vi "PicoScope6000AdvancedTriggerSettings.vi"(0 "handle in":i16, 1 "Channel A Trigger Properties":T1={"thresholdUpper"=0, "thresholdUpperHysteresis"=0, "thresholdLower"=0, "thresholdLowerHysteresis"=0, "Threshold Mode"=0, "Direction"=0, "Available"=TRUE} {"Direction" items=["Above / Inside", "Below / Outside", "Rising / Enter", "Falling / Exit", "Rising or Falling / Enter or Exit", "Above Lower", "Below Lower", "Rising Lower", "Falling Lower", "Positive Runt", "Negative Runt"]; "Threshold Mode" items=["Level", "Window"]}, 2 "Channel B Trigger Properties":T1={"thresholdUpper"=0, "thresholdUpperHysteresis"=0, "thresholdLower"=0, "thresholdLowerHysteresis"=0, "Threshold Mode"=0, "Direction"=0, "Available"=TRUE} {"Direction" items=["Above / Inside", "Below / Outside", "Rising / Enter", "Falling / Exit", "Rising or Falling / Enter or Exit", "Above Lower", "Below Lower", "Rising Lower", "Falling Lower", "Positive Runt", "Negative Runt"]; "Threshold Mode" items=["Level", "Window"]}, 3 "Channel C Trigger Properties":T1 {"Direction" items=["Above / Inside", "Below / Outside", "Rising / Enter", "Falling / Exit", "Rising or Falling / Enter or Exit", "Above Lower", "Below Lower", "Rising Lower", "Falling Lower", "Positive Runt", "Negative Runt"]; "Threshold Mode" items=["Level", "Window"]}, 5 "Auto Trigger (ms)":i32, 7 "Trigger Conditions":T4 {"Condition Logic" items=["AND", "OR", "XOR"]}, 8 "Pulse Width Qualifier Settings":T2={"Direction"=2, "Lower Limit"=0, "Upper Limit"=0, "Pulse Width Type"=4} {"Pulse Width Type" items=["None", "Less Than", "Greater Than", "In Range", "Out of Range"]; "Direction" items=["Rising"=2, "Falling"=3, "Rising Lower"=7, "Falling Lower"=8]}, 9 "Trigger Delay":u32, 10 "Pulse Width Qualifier Conditions":T3 {"Condition Logic" items=["AND", "OR", "XOR"]}, 11 "error in":errorcluster, 12 "Channel D Trigger Properties":T1 {"Direction" items=["Above / Inside", "Below / Outside", "Rising / Enter", "Falling / Exit", "Rising or Falling / Enter or Exit", "Above Lower", "Below Lower", "Rising Lower", "Falling Lower", "Positive Runt", "Negative Runt"]; "Threshold Mode" items=["Level", "Window"]}, 13 "Ext. Trigger Properties":T1 {"Direction" items=["Above / Inside", "Below / Outside", "Rising / Enter", "Falling / Exit", "Rising or Falling / Enter or Exit", "Above Lower", "Below Lower", "Rising Lower", "Falling Lower", "Positive Runt", "Negative Runt"]; "Threshold Mode" items=["Level", "Window"]}, 14 "Aux. Trigger Properties":T1 {"Direction" items=["Above / Inside", "Below / Outside", "Rising / Enter", "Falling / Exit", "Rising or Falling / Enter or Exit", "Above Lower", "Below Lower", "Rising Lower", "Falling Lower", "Positive Runt", "Negative Runt"]; "Threshold Mode" items=["Level", "Window"]}) -> (4 "handle out":i16, 15 "error out":errorcluster)   [LabVIEW 2010]
doc: "This VI is an interface for the advanced trigger features of the oscilloscope (a simple trigger can be set using PicoScope4000Settings.vi, in which case it is not necessary to use this VI)."
uses:
  ps6000.dll
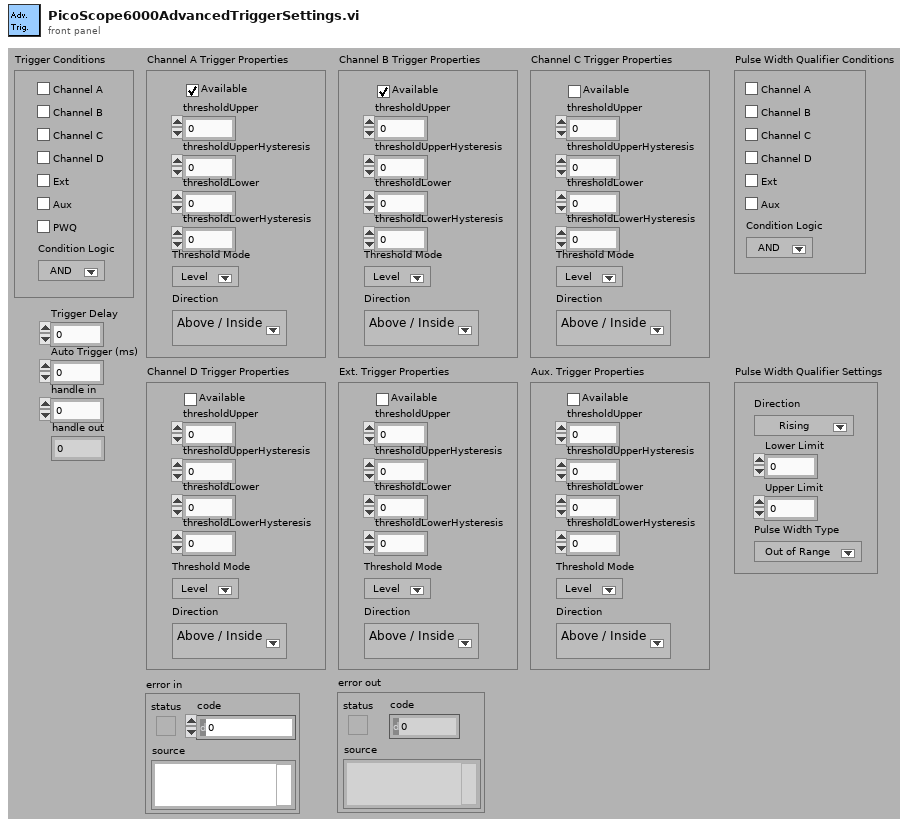
[diagram p1: front panel]
types:
  T1 = cluster{"thresholdUpper":i16, "thresholdUpperHysteresis":u16, "thresholdLower":i16, "thresholdLowerHysteresis":u16, "Threshold Mode":i32, "Direction":i32, "Available":bool}
  T2 = cluster{"Direction":i32, "Lower Limit":u32, "Upper Limit":u32, "Pulse Width Type":i32}
  T3 = cluster{"Channel A":bool, "Channel B":bool, "Channel C":bool, "Channel D":bool, "Aux":bool, "Condition Logic":u16, "Ext":bool}
  T4 = cluster{"Channel A":bool, "Channel B":bool, "Channel C":bool, "Channel D":bool, "Aux":bool, "PWQ":bool, "Condition Logic":u16, "Ext":bool}
  T5 = cluster{"thresholdUpper":i16, "thresholdUpperHysteresis":u16, "thresholdLower":i16, "thresholdLowerHysteresis":u16, "Threshold Mode":i32, "Direction":i32, "Available":bool}[]
  T6 = cluster{"[0]":i32, "[1]":i32, "[2]":i32, "[3]":i32, "[4]":i32, "[5]":i32, "[6]":i32, "[7]":i32, "[8]":i32}
  T7 = cluster{"status":bool, "code":u32, "source":string}
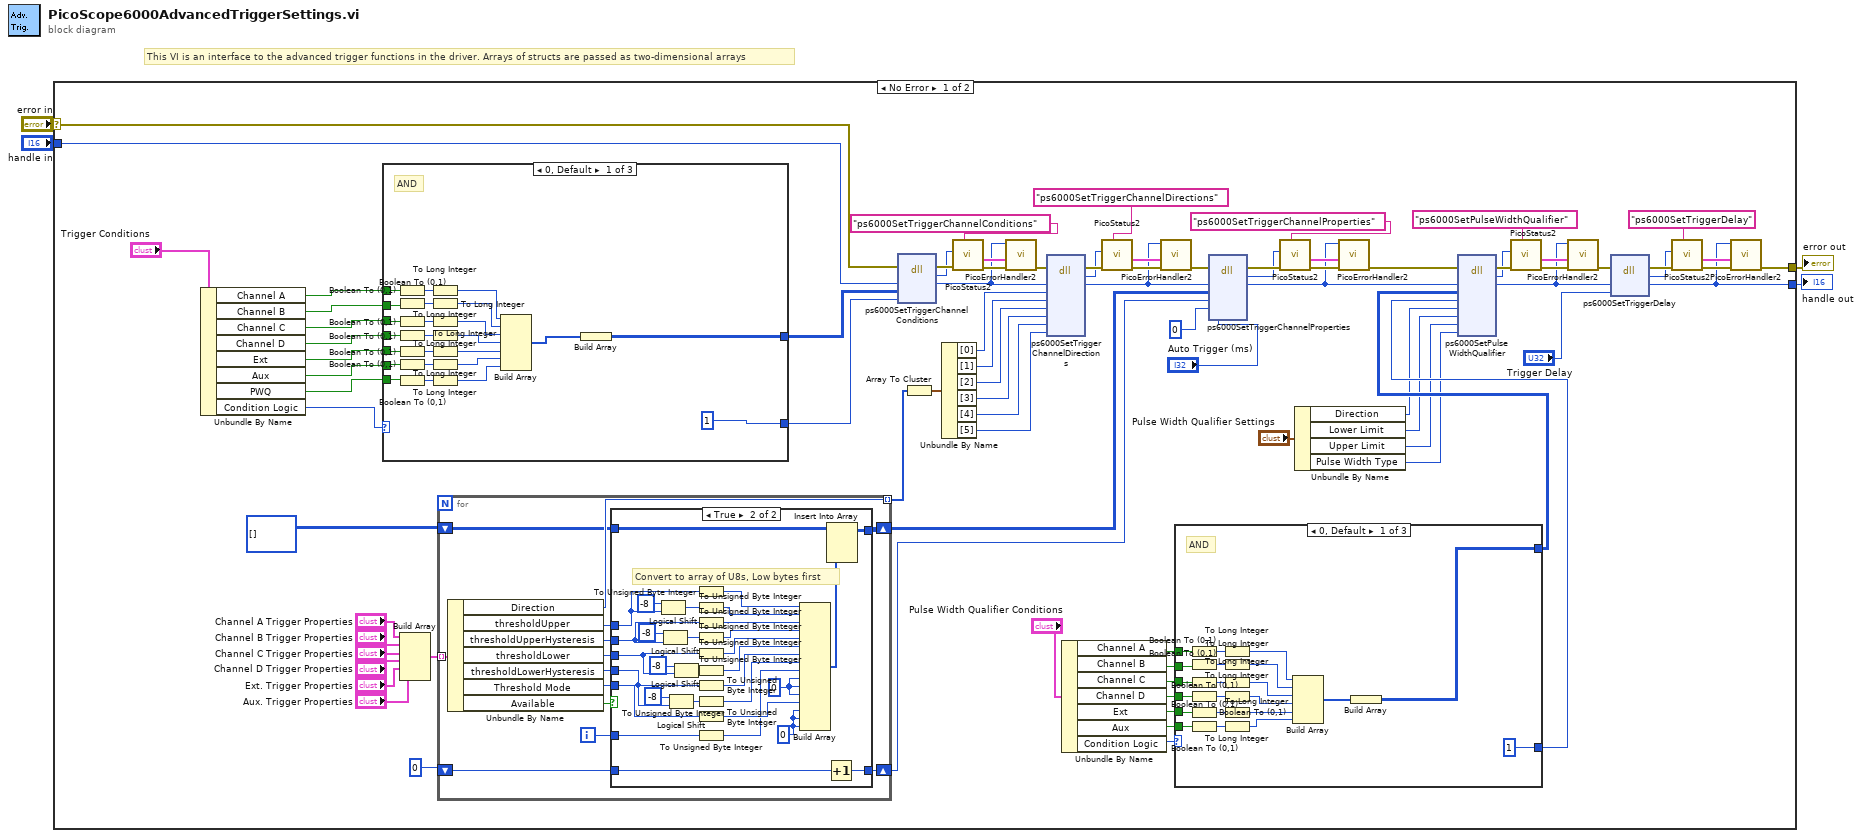
[diagram p0: block diagram]
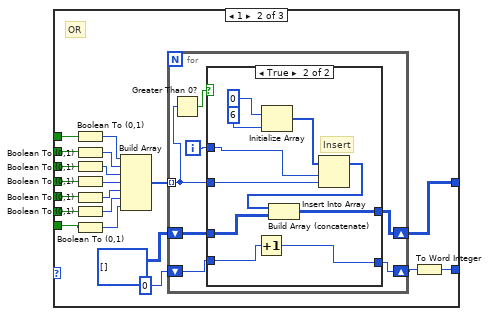
[diagram p2: hidden frame]
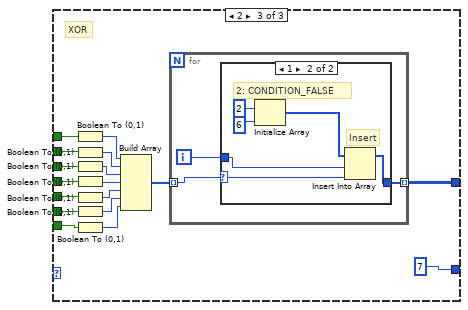
[diagram p4: hidden frame]
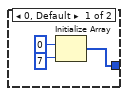
[diagram p5: hidden frame]
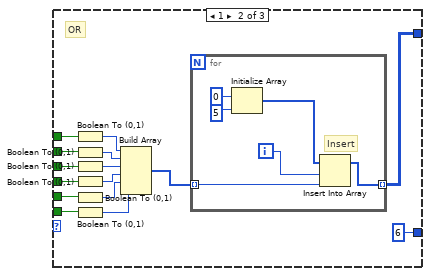
[diagram p6: hidden frame]
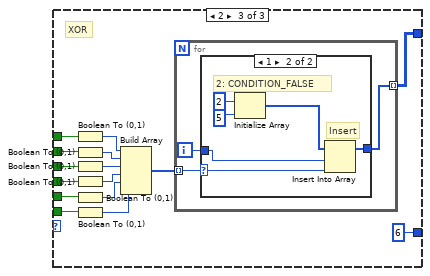
[diagram p7: hidden frame]
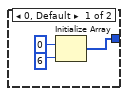
[diagram p8: hidden frame]
diagram:
  # "This VI is an interface to the advanced trigger functions in the driver. Arrays of structs are passed as two-dimensional arrays"
  n1 = case shown="No Error" "error in" {
    selector: "error in" -> [w54 w297]
    tunnel: "handle in" -> [w55 w298]
    tunnel: [w35 w298] -> w2
    tunnel: [w36 w297] -> w1
    frame No Error {
      n2 = Unbundle By Name("Trigger Conditions") -> ("Channel A"=w49:bool, "Channel B"=w48:bool, "Channel C"=w47:bool, "Channel D"=w46:bool, "Ext"=w45:bool, "Aux"=w44:bool, "PWQ"=w43:bool, "Condition Logic"=w40:u16)
      n3 = case shown="0, Default" w40 {
        tunnel: w49 -> [w113 w133 w169]
        tunnel: w48 -> [w105 w132 w168]
        tunnel: w47 -> [w104 w131 w167]
        tunnel: w46 -> [w103 w130 w166]
        tunnel: w45 -> [w102 w129 w165]
        tunnel: w44 -> [w101 w128 w164]
        tunnel: [w92 w119 w155] -> w41
        tunnel: [i16 1 w115 i16 7] -> w42
        tunnel: w43 -> [w90 w116 w153]
        frame 0, Default {
          # "AND"
          n4 = Boolean To (0,1)(Boolean=w113) -> (0, 1=w112:i16)
          n5 = Boolean To (0,1)(Boolean=w105) -> (0, 1=w111:i16)
          n6 = Boolean To (0,1)(Boolean=w104) -> (0, 1=w110:i16)
          n7 = Boolean To (0,1)(Boolean=w103) -> (0, 1=w109:i16)
          n8 = Boolean To (0,1)(Boolean=w102) -> (0, 1=w108:i16)
          n9 = Boolean To (0,1)(Boolean=w101) -> (0, 1=w107:i16)
          n10 = Boolean To (0,1)(Boolean=w90) -> (0, 1=w106:i16)
          n11 = To Long Integer(number=w112) -> (32bit integer=w100:i32)
          n12 = To Long Integer(number=w111) -> (32bit integer=w99:i32)
          n13 = To Long Integer(number=w110) -> (32bit integer=w98:i32)
          n14 = To Long Integer(number=w109) -> (32bit integer=w97:i32)
          n15 = To Long Integer(number=w108) -> (32bit integer=w96:i32)
          n16 = To Long Integer(number=w107) -> (32bit integer=w95:i32)
          n17 = To Long Integer(number=w106) -> (32bit integer=w94:i32)
          n18 = Build Array(w100, w99, w98, w97, w96, w95, w94) -> (w93:i32[])
          n19 = Build Array(w93) -> (w92:i32[][])
        }
        frame 1 {
          # "OR"
          n20 = Boolean To (0,1)(Boolean=w133) -> (0, 1=w121:i16)
          n21 = Boolean To (0,1)(Boolean=w132) -> (0, 1=w122:i16)
          n22 = Boolean To (0,1)(Boolean=w131) -> (0, 1=w123:i16)
          n23 = Boolean To (0,1)(Boolean=w130) -> (0, 1=w124:i16)
          n24 = Boolean To (0,1)(Boolean=w129) -> (0, 1=w125:i16)
          n25 = Boolean To (0,1)(Boolean=w128) -> (0, 1=w126:i16)
          n26 = Boolean To (0,1)(Boolean=w116) -> (0, 1=w127:i16)
          n27 = Build Array(w121, w122, w123, w124, w125, w126, w127) -> (w120:i16[])
          n28 = for {
            tunnel: w120 -> [w137] mode=indexing
            shift-right: [w136] -> w119
            shift-left: i32[][] [] -> [w140]
            shift-right: [w134] -> w114
            shift-left: 0 -> [w135]
            i -> [w139]
            n29 = Greater Than 0?(x=w137) -> (x > 0?=w138:bool)
            n30 = case shown="True" w138 {
              tunnel: w140 -> [w142 w145]
              tunnel: w139 -> [_ w149]
              tunnel: w137 -> [_ w148]
              tunnel: [w142 w147] -> w136
              tunnel: w135 -> [w141 w144]
              tunnel: [w141 w143] -> w134
              frame False {
              }
              frame True {
                # "Insert"
                n31 = Increment(x=w144) -> (x+1=w143:i32)
                n32 = Initialize Array(0 ("element"), 6 ("dimension size")) -> (w150:i32[])
                n33 = Insert Into Array(array=w150, index=w149, new element=w148) -> (w146:i32[])
                n34 = Build Array (concatenate)(w146, w145) -> (w147:i32[][])
              }
            }
          }
          n35 = To Word Integer(number=w114) -> (16bit integer=w115:i16)
        }
        frame 2 {
          # "XOR"
          n36 = Boolean To (0,1)(Boolean=w169) -> (0, 1=w157:i16)
          n37 = Boolean To (0,1)(Boolean=w168) -> (0, 1=w158:i16)
          n38 = Boolean To (0,1)(Boolean=w167) -> (0, 1=w159:i16)
          n39 = Boolean To (0,1)(Boolean=w166) -> (0, 1=w160:i16)
          n40 = Boolean To (0,1)(Boolean=w165) -> (0, 1=w161:i16)
          n41 = Boolean To (0,1)(Boolean=w164) -> (0, 1=w162:i16)
          n42 = Boolean To (0,1)(Boolean=w153) -> (0, 1=w163:i16)
          n43 = Build Array(w157, w158, w159, w160, w161, w162, w163) -> (w156:i16[])
          n44 = for {
            tunnel: w156 -> [w170] mode=indexing
            tunnel: [w172] -> w155 mode=indexing
            i -> [w171]
            n45 = case shown="1" w170 {
              selector: w170 -> [_ w177]
              tunnel: [w173 w178] -> w172
              tunnel: w171 -> [_ w176]
              frame 0, Default {
                n46 = Initialize Array(0 ("element"), 7 ("dimension size")) -> (w173:i32[])
              }
              frame 1 {
                # "2: CONDITION_FALSE"
                # "Insert"
                n47 = Initialize Array(2 ("element"), 6 ("dimension size")) -> (w179:i32[])
                n48 = Insert Into Array(array=w179, index=w176, new element=w177) -> (w178:i32[])
              }
            }
          }
        }
      }
      n49 = Build Array("Channel A Trigger Properties", "Channel B Trigger Properties", "Channel C Trigger Properties", "Channel D Trigger Properties", "Ext. Trigger Properties", "Aux. Trigger Properties") -> (w85:T5)
      n50 = for {
        tunnel: w85 -> [w258] mode=indexing
        tunnel: [w257] -> w84 mode=indexing
        shift-right: [w254] -> w52
        shift-left: i16 0 -> [w253]
        shift-right: [w251] -> w50
        shift-left: u8[][] [] -> [w252]
        i -> [w255]
        n51 = Unbundle By Name(w258) -> ("Direction"=w257:i32, "thresholdUpper"=w263:i16, "thresholdUpperHysteresis"=w262:u16, "thresholdLower"=w261:i16, "thresholdLowerHysteresis"=w260:u16, "Threshold Mode"=w259:i32, "Available"=w256:bool)
        n52 = case shown="True" w256 {
          tunnel: w263 -> [_ w295]
          tunnel: w262 -> [_ w287]
          tunnel: w261 -> [_ w286]
          tunnel: w260 -> [_ w285]
          tunnel: w259 -> [_ w276]
          tunnel: w255 -> [_ w271]
          tunnel: [w265 w270] -> w254
          tunnel: w253 -> [w265 w269]
          tunnel: [w264 w267] -> w251
          tunnel: w252 -> [w264 w266]
          frame False {
          }
          frame True {
            w274 = u8 0 ("element")
            w275 = u8 0 ("element")
            # "Convert to array of U8s, Low bytes first"
            n53 = Logical Shift(y=i16 -8, x=w295) -> (x << y=w294:i16)
            n54 = Logical Shift(y=i16 -8, x=w287) -> (x << y=w293:u16)
            n55 = Logical Shift(y=i16 -8, x=w285) -> (x << y=w289:u16)
            n56 = Logical Shift(y=i16 -8, x=w286) -> (x << y=w290:i16)
            n57 = To Unsigned Byte Integer(number=w295) -> (unsigned 8bit integer=w284:u8)
            n58 = To Unsigned Byte Integer(number=w294) -> (unsigned 8bit integer=w283:u8)
            n59 = To Unsigned Byte Integer(number=w287) -> (unsigned 8bit integer=w282:u8)
            n60 = To Unsigned Byte Integer(number=w293) -> (unsigned 8bit integer=w281:u8)
            n61 = To Unsigned Byte Integer(number=w286) -> (unsigned 8bit integer=w280:u8)
            n62 = To Unsigned Byte Integer(number=w290) -> (unsigned 8bit integer=w279:u8)
            n63 = To Unsigned Byte Integer(number=w285) -> (unsigned 8bit integer=w278:u8)
            n64 = To Unsigned Byte Integer(number=w289) -> (unsigned 8bit integer=w277:u8)
            n65 = To Unsigned Byte Integer(number=w276) -> (unsigned 8bit integer=w273:u8)
            n66 = To Unsigned Byte Integer(number=w271) -> (unsigned 8bit integer=w272:u8)
            n67 = Build Array(w284, w283, w282, w281, w280, w279, w278, w277, w272, w275, w275, w275, w273, w274, w274, w274) -> (w268:u8[])
            n68 = Increment(x=w269) -> (x+1=w270:i16)
            n69 = Insert Into Array(array=w266, new element=w268) -> (w267:u8[][])  [unwired: 2 in]
          }
        }
      }
      n70 = dll-call lib="PS6000.dll" fn="ps6000SetTriggerChannelConditions" ("ps3000.dll:_ps3000_open_unit@0")(error in=w54, "handle"=w55, "conditions"=w41, "nConditions"=w42) -> (error out=w20:errorcluster, "PICO_STATUS"=w9:u32, "handle"=w10:i16)  [unwired: 4 in, 1 out]
      n71 = Array To Cluster(array=w84) -> (cluster=w83:T6)
      n72 = Unbundle By Name(w83) -> ("[0]"=w82:i32, "[1]"=w81:i32, "[2]"=w80:i32, "[3]"=w79:i32, "[4]"=w78:i32, "[5]"=w77:i32)
      n73 = call "PicoStatus2.vi"("PICO source"="ps6000SetTriggerChannelConditions" ("source"), "Error in"=w20, "PICO STATUS"=w9) -> ("error out"=w22:errorcluster, "PICO_STATUS out"=w21:T7)  [unwired: 5 in]
      n74 = call "PicoErrorHandler2.vi"("error in (no error)"=w22, "PICO_STATUS in"=w21, "handle In"=w10) -> ("error out"=w19:errorcluster)  [unwired: 8 in]
      n75 = dll-call lib="PS6000.dll" fn="ps6000SetTriggerChannelDirections" ("ps3000.dll:_ps3000_open_unit@0")(error in=w19, "handle"=w10, "channelA"=w82, "channelB"=w81, "channelC"=w80, "channelD"=w79, "ext"=w78, "aux"=w77) -> (error out=w18:errorcluster, "PICO_STATUS"=w11:u32, "handle"=w12:i16)  [unwired: 8 in, 1 out]
      n76 = Unbundle By Name("Pulse Width Qualifier Conditions") -> ("Channel A"=w74:bool, "Channel B"=w73:bool, "Channel C"=w72:bool, "Channel D"=w71:bool, "Ext"=w70:bool, "Aux"=w61:bool, "Condition Logic"=w62:u16)
      n77 = call "PicoStatus2.vi"("PICO source"="ps6000SetTriggerChannelDirections" ("source"), "Error in"=w18, "PICO STATUS"=w11) -> ("error out"=w24:errorcluster, "PICO_STATUS out"=w23:T7)  [unwired: 5 in]
      n78 = call "PicoErrorHandler2.vi"("error in (no error)"=w24, "PICO_STATUS in"=w23, "handle In"=w12) -> ("error out"=w17:errorcluster)  [unwired: 8 in]
      n79 = case shown="0, Default" w62 {
        tunnel: w74 -> [w202 w217 w238]
        tunnel: w73 -> [w196 w216 w237]
        tunnel: w72 -> [w195 w215 w236]
        tunnel: w71 -> [w194 w214 w235]
        tunnel: w70 -> [w193 w205 w226]
        tunnel: [w186 w207 w228] -> w69
        tunnel: [i16 1 i16 6 i16 6] -> w68
        tunnel: w61 -> [w183 w204 w225]
        frame 0, Default {
          # "AND"
          n80 = Boolean To (0,1)(Boolean=w202) -> (0, 1=w201:i16)
          n81 = Boolean To (0,1)(Boolean=w196) -> (0, 1=w200:i16)
          n82 = Boolean To (0,1)(Boolean=w195) -> (0, 1=w199:i16)
          n83 = Boolean To (0,1)(Boolean=w194) -> (0, 1=w198:i16)
          n84 = Boolean To (0,1)(Boolean=w193) -> (0, 1=w197:i16)
          n85 = Boolean To (0,1)(Boolean=w183) -> (0, 1=w184:i16)
          n86 = To Long Integer(number=w201) -> (32bit integer=w192:i32)
          n87 = To Long Integer(number=w200) -> (32bit integer=w191:i32)
          n88 = To Long Integer(number=w199) -> (32bit integer=w190:i32)
          n89 = To Long Integer(number=w198) -> (32bit integer=w189:i32)
          n90 = To Long Integer(number=w197) -> (32bit integer=w188:i32)
          n91 = To Long Integer(number=w184) -> (32bit integer=w182:i32)
          n92 = Build Array(w192, w191, w190, w189, w188, w182) -> (w187:i32[])
          n93 = Build Array(w187) -> (w186:i32[][])
        }
        frame 1 {
          # "OR"
          n94 = Boolean To (0,1)(Boolean=w217) -> (0, 1=w209:i16)
          n95 = Boolean To (0,1)(Boolean=w216) -> (0, 1=w210:i16)
          n96 = Boolean To (0,1)(Boolean=w215) -> (0, 1=w211:i16)
          n97 = Boolean To (0,1)(Boolean=w214) -> (0, 1=w212:i16)
          n98 = Boolean To (0,1)(Boolean=w205) -> (0, 1=w213:i16)
          n99 = Boolean To (0,1)(Boolean=w204) -> (0, 1=w203:i16)
          n100 = Build Array(w209, w210, w211, w212, w213, w203) -> (w208:i16[])
          n101 = for {
            tunnel: w208 -> [w219] mode=indexing
            tunnel: [w218] -> w207 mode=indexing
            i -> [w220]
            # "Insert"
            n102 = Initialize Array(0 ("element"), 5 ("dimension size")) -> (w221:i32[])
            n103 = Insert Into Array(array=w221, index=w220, new element=w219) -> (w218:i32[])
          }
        }
        frame 2 {
          # "XOR"
          n104 = Boolean To (0,1)(Boolean=w238) -> (0, 1=w230:i16)
          n105 = Boolean To (0,1)(Boolean=w237) -> (0, 1=w231:i16)
          n106 = Boolean To (0,1)(Boolean=w236) -> (0, 1=w232:i16)
          n107 = Boolean To (0,1)(Boolean=w235) -> (0, 1=w233:i16)
          n108 = Boolean To (0,1)(Boolean=w226) -> (0, 1=w234:i16)
          n109 = Boolean To (0,1)(Boolean=w225) -> (0, 1=w224:i16)
          n110 = Build Array(w230, w231, w232, w233, w234, w224) -> (w229:i16[])
          n111 = for {
            tunnel: w229 -> [w241] mode=indexing
            tunnel: [w239] -> w228 mode=indexing
            i -> [w240]
            n112 = case shown="1" w241 {
              selector: w241 -> [_ w246]
              tunnel: [w242 w247] -> w239
              tunnel: w240 -> [_ w245]
              frame 0, Default {
                n113 = Initialize Array(0 ("element"), 6 ("dimension size")) -> (w242:i32[])
              }
              frame 1 {
                # "2: CONDITION_FALSE"
                # "Insert"
                n114 = Initialize Array(2 ("element"), 5 ("dimension size")) -> (w248:i32[])
                n115 = Insert Into Array(array=w248, index=w245, new element=w246) -> (w247:i32[])
              }
            }
          }
        }
      }
      n116 = dll-call lib="PS6000.dll" fn="ps6000SetTriggerChannelProperties" ("ps3000.dll:_ps3000_open_unit@0")(error in=w17, "handle"=w12, "channelProperties"=w50, "nChannelProperties"=w52, "auxOutputEnable"=i16 0, "autoTriggerMilliseconds"="Auto Trigger (ms)") -> (error out=w15:errorcluster, "PICO_STATUS"=w13:u32, "handle"=w14:i16)  [unwired: 6 in, 1 out]
      n117 = call "PicoStatus2.vi"("PICO source"="ps6000SetTriggerChannelProperties" ("source"), "Error in"=w15, "PICO STATUS"=w13) -> ("error out"=w26:errorcluster, "PICO_STATUS out"=w25:T7)  [unwired: 5 in]
      n118 = Unbundle By Name("Pulse Width Qualifier Settings") -> ("Direction"=w66:i32, "Lower Limit"=w65:u32, "Upper Limit"=w64:u32, "Pulse Width Type"=w63:i32)
      n119 = call "PicoErrorHandler2.vi"("error in (no error)"=w26, "PICO_STATUS in"=w25, "handle In"=w14) -> ("error out"=w16:errorcluster)  [unwired: 8 in]
      n120 = dll-call lib="PS6000.dll" fn="ps6000SetPulseWidthQualifier" ("ps3000.dll:_ps3000_open_unit@0")(error in=w16, "handle"=w14, "conditions"=w69, "nConditions"=w68, "direction"=w66, "lower"=w65, "upper"=w64, "type"=w63) -> (error out=w30:errorcluster, "PICO_STATUS"=w27:u32, "handle"=w28:i16)  [unwired: 8 in, 1 out]
      n121 = call "PicoStatus2.vi"("PICO source"="ps6000SetPulseWidthQualifier" ("source"), "Error in"=w30, "PICO STATUS"=w27) -> ("error out"=w32:errorcluster, "PICO_STATUS out"=w31:T7)  [unwired: 5 in]
      n122 = call "PicoErrorHandler2.vi"("error in (no error)"=w32, "PICO_STATUS in"=w31, "handle In"=w28) -> ("error out"=w29:errorcluster)  [unwired: 8 in]
      n123 = dll-call lib="ps6000.dll" fn="ps6000SetTriggerDelay" ("ps3000.dll:_ps3000_open_unit@0")(error in=w29, "handle"=w28, "delay"="Trigger Delay") -> (error out=w37:errorcluster, "PICO_STATUS"=w34:u32, "handle"=w35:i16)  [unwired: 3 in, 1 out]
      n124 = call "PicoStatus2.vi"("PICO source"="ps6000SetTriggerDelay" ("source"), "Error in"=w37, "PICO STATUS"=w34) -> ("error out"=w39:errorcluster, "PICO_STATUS out"=w38:T7)  [unwired: 5 in]
      n125 = call "PicoErrorHandler2.vi"("error in (no error)"=w39, "PICO_STATUS in"=w38, "handle In"=w35) -> ("error out"=w36:errorcluster)  [unwired: 8 in]
    }
    frame Error {
    }
  }
  "handle out" <- w2
  "error out" <- w1
